vi "trace_extra.vi"(1 "Extra trace data":sgl[](array[numeric])) -> ()   [LabVIEW 2013]
panel:
  # "Supply data to be added to the trace in the \"Trace data 0\", \"Trace data 1\".   Data is reshaped to be a 6-vector."
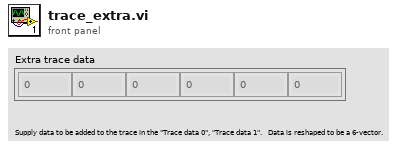
[diagram p1: front panel]
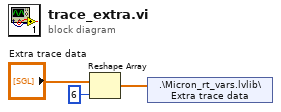
[diagram p0: block diagram]
diagram:
  n1 = Reshape Array("Extra trace data", 6 ("dimension size")) -> (w1:sgl[])
  n2 = shared-variable ".\\Micron_rt_vars.lvlib\\Extra trace data"(w1) -> ()  [unwired: 2 out]
